vi "Do.vi"(8 "error in (no error)":errorcluster, 11 "Proto in":refnum<class "Proto.lvclass">) -> (0 "error out":errorcluster, 2 "set":set{set{string}}(c389), 3 "Proto out":refnum<class "Proto.lvclass">)   [LabVIEW 2020, in "Proto.lvclass"]
uses:
  Proto.lvclass
  Proto.lvclass/Proto.ctl
  5dd8e771-5231-4cab-83dc-df207e51e12b.vi
panel:
  out "Array":i32[](array[numeric])
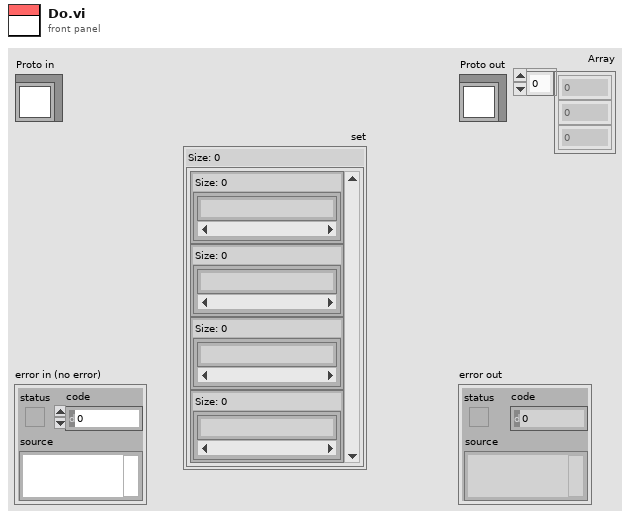
[diagram p1: front panel]
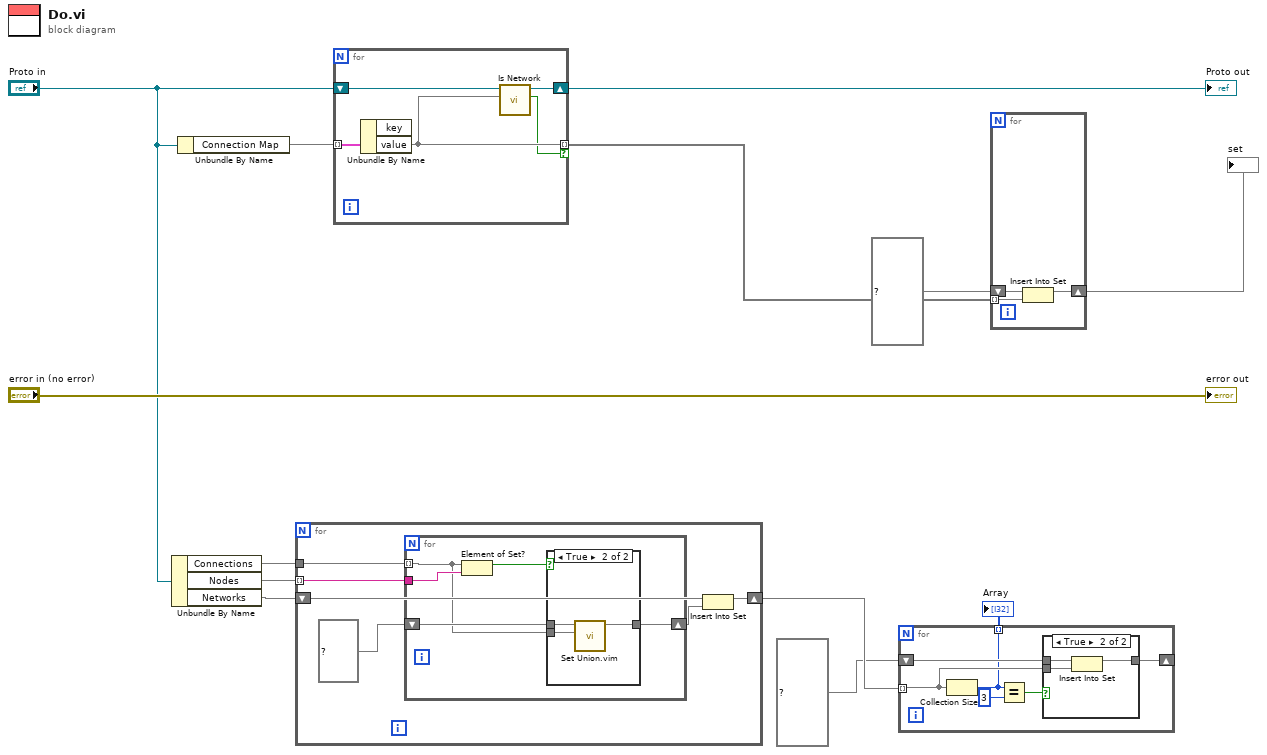
[diagram p0: block diagram]
diagram:
  n1 = Unbundle By Name("Proto in") -> ("Connections"=w11:set{set{string}}, "Nodes"=w12:set{string}, "Networks"=w10:set{set{string}})
  n2 = Unbundle By Name("Proto in") -> ("Connection Map"=w6:map{string, set{string}})
  n3 = for {
    tunnel: w12 -> [w18] mode=indexing
    tunnel: w11 -> [w19]
    shift-right: [w16] -> w9
    shift-left: w10 -> [w15]
    n4 = for {
      tunnel: w19 -> [w22] mode=indexing
      tunnel: w18 -> [w24]
      shift-right: [w21] -> w14
      shift-left: set{string} {} ("set") -> [w23]
      n5 = Element of Set?(10:w24, 11:w22) -> (3:w20:bool)
      n6 = case shown="True" w20 {
        tunnel: w23 -> [w25 w28]
        tunnel: w22 -> [_ w27]
        tunnel: [w25 w26] -> w21
        frame False {
        }
        frame True {
          n7 = call "Set Union.vim"("set 2"=w27, "set 1"=w28) -> ("union"=w26:set{string})  [unwired: 9 in]
        }
      }
    }
    n8 = Insert Into Set(10:w14, 11:w15) -> (3:w16:set{set{string}})  [unwired: 1 out]
  }
  n9 = for {
    tunnel: w6 -> [w33] mode=indexing
    tunnel: [w32] -> w3 mode=indexing if=w31
    shift-right: [w29] -> w1
    shift-left: "Proto in" -> [w30]
    n10 = Unbundle By Name(w33) -> ("value"=w32:set{string})  [unwired: 1 out]
    n11 = call "Is Network.vi"("Connection"=w32, "Proto in"=w30) -> ("nerwork?"=w31:bool, "Proto out"=w29:refnum<class "Proto.lvclass">)  [unwired: 8 in]
  }
  "Proto out" <- w1
  n12 = for {
    tunnel: w9 -> [w35] mode=indexing
    shift-right: [w38] -> _
    shift-left: set{set{string}} {} ("Networks") -> [w39]
    tunnel: [w34] -> w7 mode=indexing
    n13 = Collection Size(1:w35) -> (0:w34:i32)
    n14 = Equal?(x=w34, y=3) -> (x = y?=w36:bool)
    n15 = case shown="True" w36 {
      tunnel: w39 -> [w40 w43]
      tunnel: [w40 w42] -> w38
      tunnel: w35 -> [_ w41]
      frame False {
      }
      frame True {
        n16 = Insert Into Set(10:w41, 11:w43) -> (3:w42:set{set{string}})  [unwired: 1 out]
      }
    }
  }
  "Array" <- w7
  n17 = for {
    shift-right: [w45] -> w4
    shift-left: set{set{string}} {} ("set") -> [w46]
    tunnel: w3 -> [w44] mode=indexing
    n18 = Insert Into Set(10:w44, 11:w46) -> (3:w45:set{set{string}})  [unwired: 1 out]
  }
  "set" <- w4
  "error out" <- "error in (no error)"
